vi "VI Tree.vi"   [LabVIEW 2012, in "Phidget DC Motor.lvlib"]
doc: "${DCMotor:VITreeHeader}"
uses:
  <instrlib>/Phidgets/Phidget DC Motor/Phidget DC Motor.lvlib
  <instrlib>/Phidgets/Phidget DC Motor/Public/DCMotorStart.vi
  <instrlib>/Phidgets/Phidget DC Motor/Public/DCMotorOpen.vi
  <instrlib>/Phidgets/Phidget DC Motor/Public/DCMotorClose.vi
panel:
  # "(c) 2015 Phidgets Inc..  ALL RIGHTS RESERVED."
  # "SEE DIAGRAM\nFOR VI TREE."
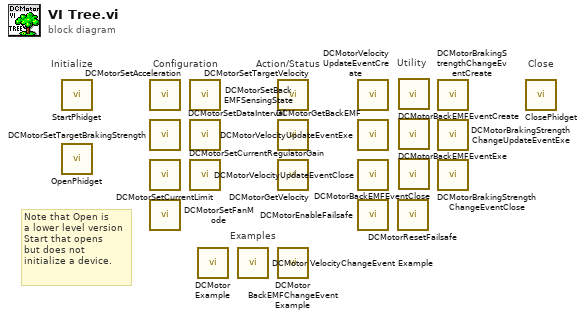
[diagram p0: block diagram]
diagram:
  # "Note that Open is\na lower level version\nStart that opens\nbut does not \ninitialize a device."
  # "Examples"
  # "Configuration"
  # "Utility"
  # "Action/Status"
  # "Close"
  # "Initialize"
  n1 = call-poly <instrlib>:"StartPhidget.vi"() -> ()  [unwired: 12 in, 4 out]
  n2 = call-poly <instrlib>:"OpenPhidget.vi"() -> ()  [unwired: 8 in, 4 out]
  n3 = call <instrlib>:"DCMotorSetAcceleration.vi"() -> ()  [unwired: 9 in, 2 out]
  n4 = call <instrlib>:"DCMotorSetTargetBrakingStrength.vi"() -> ()  [unwired: 9 in, 2 out]
  n5 = call <instrlib>:"DCMotorSetCurrentLimit.vi"() -> ()  [unwired: 9 in, 2 out]
  n6 = call <instrlib>:"DCMotorSetFanMode.vi"() -> ()  [unwired: 9 in, 2 out]
  n7 = call <instrlib>:"DCMotorSetBackEMFSensingState.vi"() -> ()  [unwired: 9 in, 2 out]
  n8 = call <instrlib>:"DCMotorSetDataInterval.vi"() -> ()  [unwired: 9 in, 2 out]
  n9 = call <instrlib>:"DCMotorSetCurrentRegulatorGain.vi"() -> ()  [unwired: 9 in, 2 out]
  n10 = call <instrlib>:"DCMotor Example.vi"() -> ()  [unwired: 12 in]
  n11 = call <instrlib>:"DCMotor VelocityChangeEvent Example.vi"() -> ()  [unwired: 12 in]
  n12 = call <instrlib>:"DCMotorSetTargetVelocity.vi"() -> ()  [unwired: 9 in, 2 out]
  n13 = call <instrlib>:"DCMotorGetBackEMF.vi"() -> ()  [unwired: 8 in, 3 out]
  n14 = call <instrlib>:"DCMotorGetVelocity.vi"() -> ()  [unwired: 8 in, 3 out]
  n15 = call <instrlib>:"DCMotor BackEMFChangeEvent Example.vi"() -> ()  [unwired: 12 in]
  n16 = call <instrlib>:"DCMotorVelocityUpdateEventCreate.vi"() -> ()  [unwired: 9 in, 3 out]
  n17 = call <instrlib>:"DCMotorVelocityUpdateEventExe.vi"() -> ()  [unwired: 5 in, 7 out]
  n18 = call <instrlib>:"DCMotorVelocityUpdateEventClose.vi"() -> ()  [unwired: 10 in, 2 out]
  n19 = call <instrlib>:"DCMotorEnableFailsafe.vi"() -> ()  [unwired: 9 in, 2 out]
  n20 = call <instrlib>:"DCMotorResetFailsafe.vi"() -> ()  [unwired: 9 in, 2 out]
  n21 = call <instrlib>:"DCMotorBackEMFEventCreate.vi"() -> ()  [unwired: 9 in, 3 out]
  n22 = call <instrlib>:"DCMotorBackEMFEventExe.vi"() -> ()  [unwired: 5 in, 7 out]
  n23 = call <instrlib>:"DCMotorBackEMFEventClose.vi"() -> ()  [unwired: 10 in, 2 out]
  n24 = call <instrlib>:"DCMotorBrakingStrengthChangeEventCreate.vi"() -> ()  [unwired: 9 in, 3 out]
  n25 = call <instrlib>:"DCMotorBrakingStrengthChangeUpdateEventExe.vi"() -> ()  [unwired: 5 in, 7 out]
  n26 = call <instrlib>:"DCMotorBrakingStrengthChangeEventClose.vi"() -> ()  [unwired: 10 in, 2 out]
  n27 = call-poly <instrlib>:"ClosePhidget.vi"() -> ()  [unwired: 11 in, 1 out]
